vi "Init Msg Default.vi"() -> (3 "Stopped Msg out":refnum<class "Stopped Msg.lvclass">)   [LabVIEW 2020, in "jettl.lvlib" / "Stopped jettl Msg.lvlib" / "Stopped Msg.lvlib" / "Stopped Msg.lvclass"]
uses:
  Stopped Msg.lvclass
  Stopped Msg.lvclass/Stopped Msg.ctl
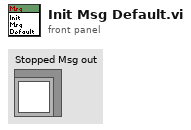
[diagram p1: front panel]
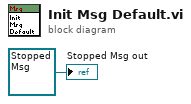
[diagram p0: block diagram]
diagram:
  "Stopped Msg out" <- refnum<class "Stopped Msg.lvclass"> refnum ("Last Ack Creator Queue Msg Strategy out")
